vi "Testbench for Helper - Overlay Waypoints.vi"() -> ()   [LabVIEW 2011]
doc: "This is a test bench for Helper - Overlay waypoints.vi. It prompts the user to open an image file, then sends that file to the sub-vi for overlaying of waypoint locations. The resultant image is displayed.\n\nPurpose: to test Helper - Overlay waypoints.vi.\n\nAuthor: Jason Curtis"
panel:
  out "Image":T1(plugin-control)
  # "WARNING: DO NOT run continuously. you will be forever prompted to open images..."
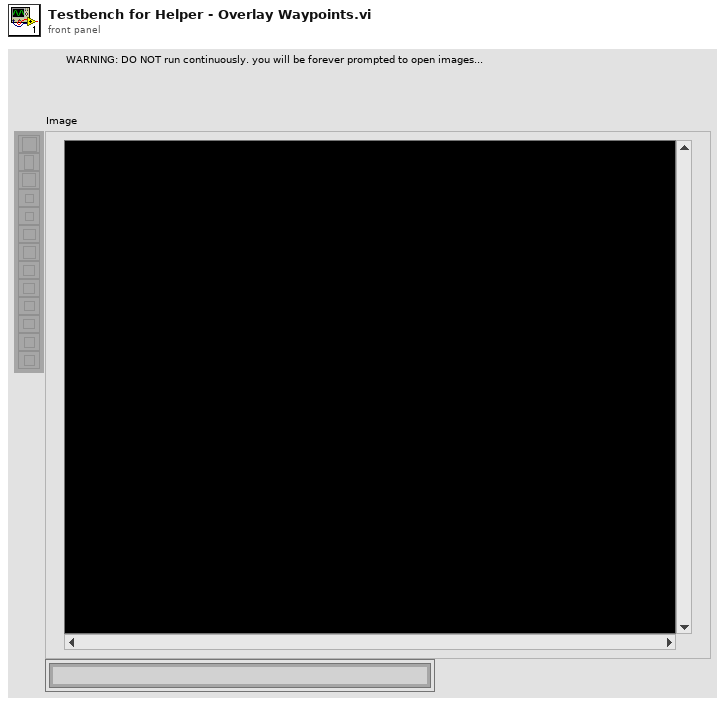
[diagram p1: front panel]
types:
  T1 = typedef "IMAQ Image.ctl" = refnum<image>
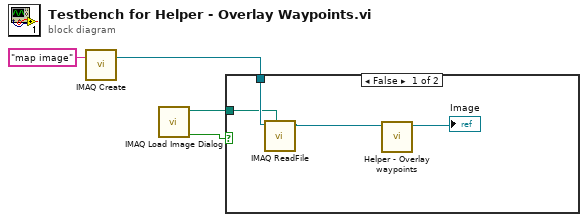
[diagram p0: block diagram]
diagram:
  n1 = call "IMAQ Create"("Image Name"="map image") -> ("New Image"=w4:T1)  [unwired: 4 in, 1 out]
  n2 = call "IMAQ Load Image Dialog"() -> ("Cancelled?"=w2:bool, "Path"=w3:path)  [unwired: 9 in, 1 out]
  n3 = case shown="False" w2 {
    tunnel: w4 -> [w7 _]
    tunnel: w3 -> [w6 _]
    frame False {
      n4 = call "IMAQ ReadFile"("File Path"=w6, "Image"=w7) -> ("Image Out"=w8:T1)  [unwired: 5 in, 4 out]
      n5 = call "Helper - Overlay waypoints.vi"("Img Refnum in"=w8) -> ("Img Refnum out"=→"Image":T1)  [unwired: 10 in]
    }
    frame True {
    }
  }
